vi "Format String.vi"(1 "Display":T1) -> (0 "format":string)   [LabVIEW 2020, in "Value.lvlib"]
uses:
  Value.lvlib
  Display Metadata.ctl
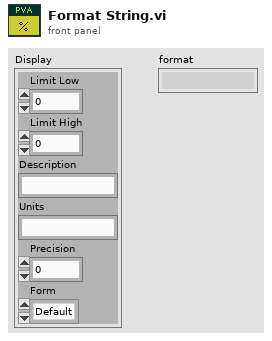
[diagram p1: front panel]
types:
  T1 = typedef "Value.lvlib/Display Metadata.ctl" = cluster{"Limit Low":dbl, "Limit High":dbl, "Description":string, "Units":string, "Precision":i32, "Form":enum32{"Default", "String", "Binary", "Decimal", "Hex", "Exponential", "Engineering"}}
  T2 = enum32{"Default", "String", "Binary", "Decimal", "Hex", "Exponential", "Engineering"}
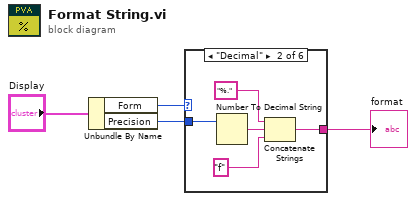
[diagram p0: block diagram]
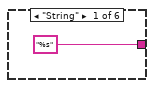
[diagram p2: hidden frame]
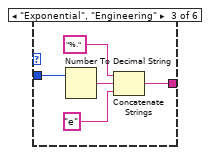
[diagram p3: hidden frame]
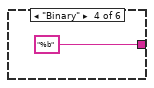
[diagram p4: hidden frame]
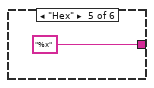
[diagram p5: hidden frame]
diagram:
  n1 = Unbundle By Name("Display") -> ("Form"=w3:T2, "Precision"=w2:i32)
  n2 = case shown="\"Decimal\"" w3 {
    tunnel: w2 -> [_ w10 w15 _ _ _]
    tunnel: ["%s" w9 w13 "%b" "%x" _] -> w1
    frame "String" {
    }
    frame "Decimal" {
      n3 = Number To Decimal String(number=w10) -> (decimal integer string=w8:string)  [unwired: 1 in]
      n4 = Concatenate Strings("%.", w8, "f") -> (w9:string)
    }
    frame "Exponential", "Engineering" {
      n5 = Number To Decimal String(number=w15) -> (decimal integer string=w12:string)  [unwired: 1 in]
      n6 = Concatenate Strings("%.", w12, "e") -> (w13:string)
    }
    frame "Binary" {
    }
    frame "Hex" {
    }
    frame Default {
    }
  }
  "format" <- w1
